vi "access.vi"(5 "Control_enum":T1, 6 "error in (no error)":errorcluster) -> (0 "error out":errorcluster, 2 "output":u32)   [LabVIEW 2023]
doc: "FGV\nUsed to solve the problem of currency access. \nIt has 3 states:\nread --> read the value stored in the register\nwrite --> write the value to the register\nclear --> value = 0"
uses:
  cntrls/control_enum.ctl
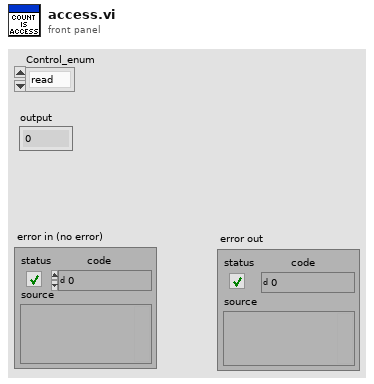
[diagram p1: front panel]
types:
  T1 = typedef "control_enum.ctl" = enum16{"read", "write", "clear"}
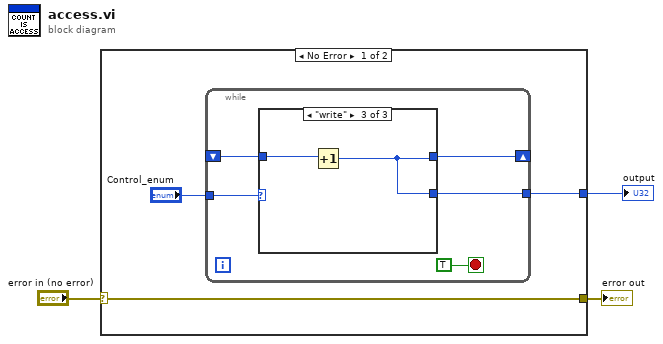
[diagram p0: block diagram]
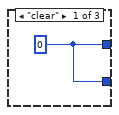
[diagram p2: hidden frame]
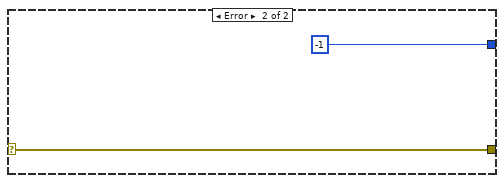
[diagram p4: hidden frame]
diagram:
  n1 = case shown="No Error" "error in (no error)" {
    selector: "error in (no error)" -> [w6 w17]
    tunnel: [w6 w17] -> w2
    tunnel: [w4 -1] -> w1
    frame No Error {
      n2 = while {
        shift-right: [w8] -> _
        shift-left: _ -> [w9]
        tunnel: "Control_enum" -> [w10]
        tunnel: [w7] -> w4
        stop <- TRUE stop-if-true
        n3 = case shown="\"write\"" w10 {
          tunnel: w9 -> [_ w13 w15]
          tunnel: [w12 w13 w14] -> w8
          tunnel: [w12 w13 w14] -> w7
          frame "clear" {
            w12 = 0
          }
          frame "read", Default {
          }
          frame "write" {
            n4 = Increment(x=w15) -> (x+1=w14:i32)
          }
        }
      }
    }
    frame Error {
    }
  }
  "error out" <- w2
  "output" <- w1
